vi "2a_ths_browser.vi"() -> ()   [LabVIEW 2020]
panel:
  out "MainImg":u16[][](graph)
  out "Th Scan":u16[](graph)=[1, 1, 1, 1, 1, 1, 1, 1, 1, 1, 1, 1, 1, 1, 1, 1, 1, 1, 1, 1, 1, 1, 1, 1, 1, 1, 1, 1, 1, 1, 1, 1, 1, 1, 1, 1, 1, 1, 1, 1, 1, 1, 1, 1, 1, 1, 1, 1, 1, 1, 1, 1, 1, 1, 1, 1, 1, 1, 1, 2, 2, 1, 2, 4, 6, 11, 22, 37, 72, 86, 151, 192, 290, 416, 520, 682, 880, 1117, 1222, 1425, 1613, 1780, 1961, 2019, 1943, 1943, 1774, 1537, 1392, 1249, 1136, 1048, 927, 788, 625, 447, 326, 215, 171, 125, 79, 50, 43, 34, 16, 11, 4, 5, 3, 1, 1, 0, 0, 0, 0, 0, 0, 0, 0, 0, 0, 0, 0, 0, 0, 0, 0, 0, 0, 0, 0, 0, 0, 0, 0, 0, 0, 0, 0, 0, 0, 0, 0, 0, 0, 0, 0, 0, 0, 0, 0, 0, 0, 0, 0, 0, 0, 0, 0, 0, 0, 0, 0, 0, 0, 0, 0, 0, 0, 0, 0, 0, 0, 0, 0, 0, 0, 0, 0, 0, 0, 0, 0, 0, 0, 0, 0, 0, 0, 0, 0, 0, 0, 0, 0, 0, 0, 0, 0, 0, 0, 0, 0, 0, 0, 0, 0, 0, 0, 0, 0, 0, 0, 0, 0, 0, 0, 0, 0, 0, 0, 0, 0, 0, 0, 0, 0, 0, 0, 0, 0, 0, 0, 0, 0, 0, 0, 0, 0, 0, 0, 0, 0, 0, 0, 0, 0, 0, 0, 0, 0, 0, 0, 0, 0, 0, 0, 0, 0, 0, 0, 0, 0, 0, 0, 0, 0, 0, 0, 0, 0, 0, 0, 0, 0, 0, 0, 0, 0, 0, 0, 0, 0, 0, 0, 0, 0, 0, 0, 0, 0, 0, 0, 0, 0, 0, 0, 0, 0, 0, 0, 0, 0, 0, 0, 0, 0, 0, 0, 0, 0, 0, 0, 0, 0, 0, 0, 0, 0, 0, 0, 0, 0, 0, 0, 0, 0, 0, 0, 0, 0, 0, 0, 0, 0, 0, 0, 0, 0, 0, 0, 0, 0, 0, 0, 0, 0, 0, 0, 0, 0, 0, 0, 0, 0, 0, 0, 0, 0, 0, 0, 0, 0, 0, 0, 0, 0, 0, 0, 0, 0, 0, 0, 0, 0, 0, 0, 0, 0, 0, 0, 0, 0, 0, 0, 0, 0, 0, 0, 0, 0, 0, 0, 0, 0, 0, 0, 0, 0, 0, 0, 0, 0, 0, 0, 0, 0, 0, 0, 0, 0, 0, 0, 0, 0, 0, 0, 0, 0, 0, 0, 0, 0, 0, 0, 0, 0, 0, 0, 0, 0, 0, 0, 0, 0, 0, 0, 0, 0, 0, 0, 0, 0, 0, 0, 0, 0, 0, 0, 0, 0, 0, 0, 0, 0, 0, 0, 0, 0, 0, 0, 0, 0, 0, 0, 0, 0, 0, 0, 0, 0, 0, 0, 0, 0, 0, 0, 0, 0, 0, 0, 0, 0, 0, 0, 0, 0, 0, 0, 0, 0, 0, 0, 0, 0, 0, 0, 0, 0, 0, 0, 0, 0, 0, 0, 0, 0, 0, 0, 0]
  in  "ThScan_Load":bool
  out "ThScan":i32[][][](array[numeric])
  in  "Exit":bool
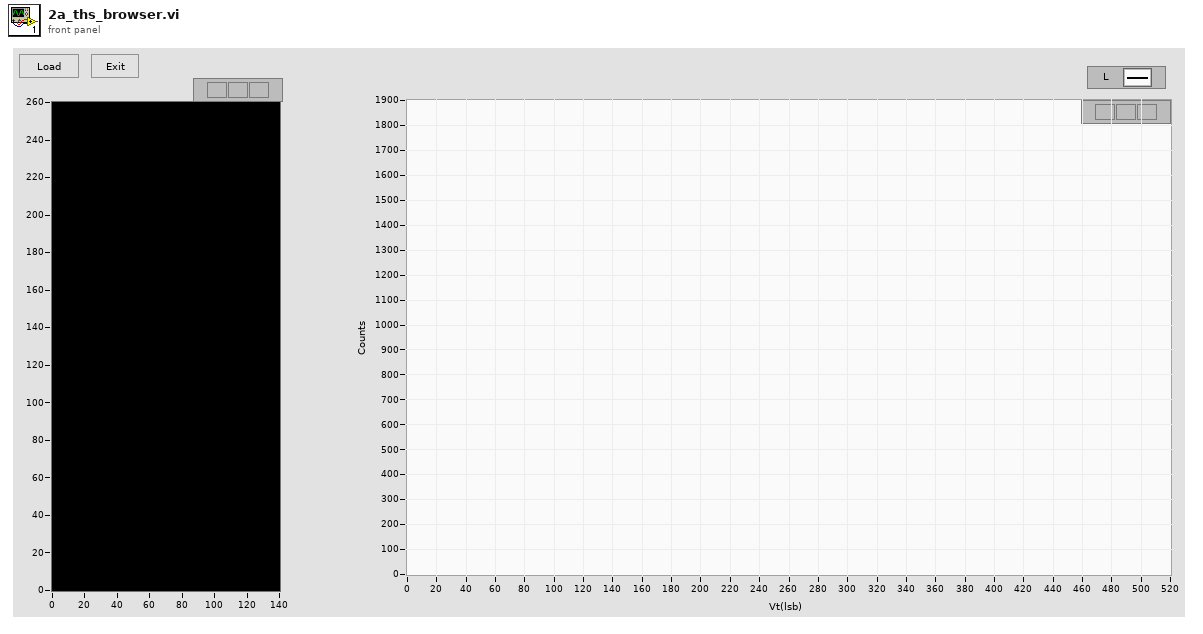
[diagram p1: front panel]
types:
  T1 = enum16{"big-endian, network order", "native, host order", "little-endian"}
  T2 = typedef "LVPointDoubleTypeDef.ctl" = cluster{"Cursor X":dbl, "Cursor Y":dbl}
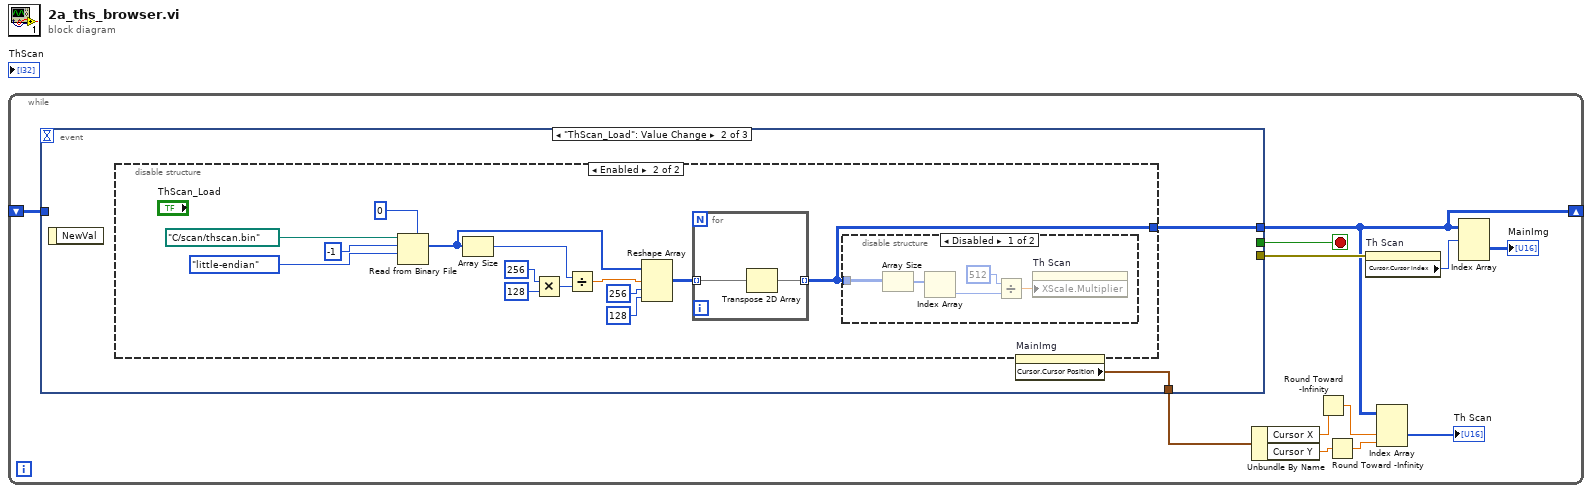
[diagram p0: block diagram]
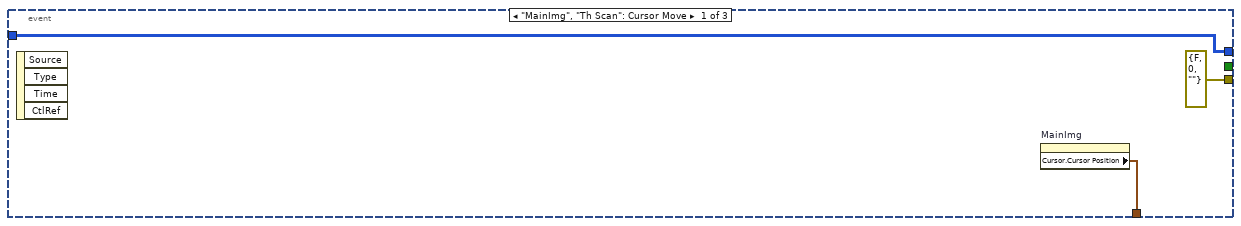
[diagram p2: hidden frame]
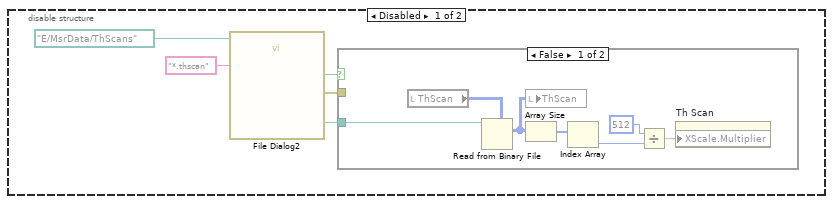
[diagram p3: hidden frame]
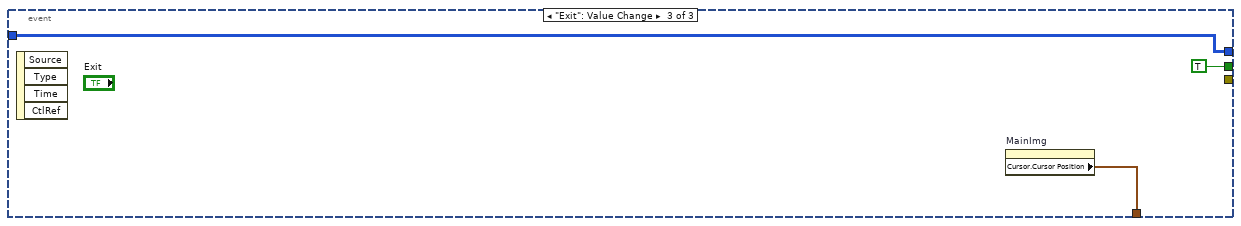
[diagram p6: hidden frame]
diagram:
  n1 = while {
    shift-right: [w7] -> _
    shift-left: _ -> [w6]
    stop <- w12 stop-if-true
    n2 = event shown="[1] \"ThScan_Load\": Value Change" {
      selector: _ -> [_ _ _]
      dyn-events: _ -> [_ _ _]
      timeout: _ -> [_ _ _]
      tunnel: [_ _ TRUE] -> w12
      tunnel: [errorcluster {"status"=FALSE, "code"=0, "source"=""} ("error in (no error)") _ _] -> w8
      tunnel: w6 -> [w14 _ w52]
      tunnel: [w14 w17 w52] -> w7
      tunnel: [w13 w16 w51] -> w3
      event "MainImg", "Th Scan": Cursor Move {
        n3 = event-data() -> ()  [unwired: 1 in, 4 out]
        n4 = property on="MainImg" class="IntGraph (strict)"() -> ("Cursor.Cursor Position"=w13:T2)  [unwired: 2 in, 2 out]
      }
      event "ThScan_Load": Value Change {
        n5 = event-data() -> ()  [unwired: 1 in, 1 out]
        n6 = disable-structure shown="Enabled" {
          disable-tunnel: [_ w30] -> w17
          frame Disabled {
            n7 = call "File Dialog2"("start path"=path "E:/MsrData/ThScans" ("Current path"), "pattern (all files)"="*.thscan") -> ("selected path"=w21:path, "cancelled"=w20:bool, "error out"=w19:errorcluster)  [unwired: 10 in, 1 out]
            n8 = case shown="False" w20 {
              tunnel: w21 -> [w29 _]
              tunnel: w19 -> [_ _]
              frame False {
                n9 = local read "ThScan"() -> (w28:i32[][][])
                n10 = Read from Binary File(5:w28, 11:w29) -> (2:w27:i32[][][])  [unwired: 4 in, 3 out]
                n11 = local write "ThScan"(w27) -> ()
                n12 = Array Size(array=w27) -> (size(s)=w26:i32[])
                n13 = Index Array(array=w26) -> (element=w25:i32)  [unwired: 1 in]
                n14 = Divide(x=512, y=w25) -> (x/y=w23:dbl)
                n15 = property on="Th Scan" class="WFGraph (strict)"("XScale.Multiplier"=w23) -> ()  [unwired: 2 in, 2 out]
              }
              frame True {
              }
            }
          }
          frame Enabled {
            n16 = Read from Binary File(5:u16 0, 9:T1."little-endian" ("byte order (0:big-endian, network order)"), 10:-1 ("count (1)"), 11:path "C:/scan/thscan.bin" ("file (use dialog)")) -> (2:w32:u16[])  [unwired: 2 in, 3 out]
            n17 = Array Size(array=w32) -> (size(s)=w37:i32)
            n18 = Multiply(x=256 ("dimension size"), y=128 ("dimension size")) -> (x*y=w34:i32)
            n19 = Divide(x=w37, y=w34) -> (x/y=w33:dbl)
            n20 = Reshape Array(w32, w33, 256 ("dimension size"), 128 ("dimension size")) -> (w31:u16[][][])
            n21 = for {
              tunnel: w31 -> [w50] mode=indexing
              tunnel: [w49] -> w30 mode=indexing
              n22 = Transpose 2D Array(2D array=w50) -> (transposed array=w49:u16[][])
            }
            n23 = disable-structure shown="Disabled" {
              disable-tunnel: w30 -> [w44 _]
              frame Disabled {
                n24 = Array Size(array=w44) -> (size(s)=w48:i32[])
                n25 = Index Array(array=w48) -> (element=w47:i32)  [unwired: 1 in]
                n26 = Divide(x=512, y=w47) -> (x/y=w45:dbl)
                n27 = property on="Th Scan" class="WFGraph (strict)"("XScale.Multiplier"=w45) -> ()  [unwired: 2 in, 2 out]
              }
              frame Enabled {
              }
            }
          }
        }
        n28 = property on="MainImg" class="IntGraph (strict)"() -> ("Cursor.Cursor Position"=w16:T2)  [unwired: 2 in, 2 out]
      }
      event "Exit": Value Change {
        n29 = event-data() -> ()  [unwired: 1 in, 4 out]
        n30 = property on="MainImg" class="IntGraph (strict)"() -> ("Cursor.Cursor Position"=w51:T2)  [unwired: 2 in, 2 out]
      }
    }
    n31 = Unbundle By Name(w3) -> ("Cursor X"=w2:dbl, "Cursor Y"=w4:dbl)
    n32 = Round Toward -Infinity(1:w2) -> (0:w1:dbl)
    n33 = Round Toward -Infinity(1:w4) -> (0:w5:dbl)
    n34 = property on="Th Scan" class="WFGraph (strict)"(error in=w8) -> ("Cursor.Cursor Index"=w9:i32)  [unwired: 1 in, 2 out]
    n35 = Index Array(array=w7, index (dim 1)=w1, index (dim 2)=w5) -> (element=→"Th Scan":u16[])  [unwired: 1 in]
    n36 = Index Array(array=w7, index (dim 0)=w9) -> (element=→"MainImg":u16[][])  [unwired: 2 in]
  }
